vi "Fetch Power Measurement List Mode.vi"(6 "Step Index (1)":i32=1, 7 "Detector Type (RMS)":i32(ring) items=["RMS", "Minimum", "Maximum"], 8 "error in (no error)":errorcluster, 9 "Result Type (Current)":i32(ring) items=["Current", "Average", "Peak"], 10 "Instance (1)":i32=1, 11 "VISA resource name":refnum<visa-resource-name>) -> (0 "error out":errorcluster, 1 "Power":dbl format="%^.3e", 2 "Reliability":i32, 3 "VISA resource name out":refnum<visa-resource-name>)   [LabVIEW 2020, in "Rohde&Schwarz CMXP GPRF.lvlib"]
doc: "Returns the results of the GPRF power measurement for single step and \"Statistic\" evaluation mode. Initiate measurement first with VI rscmwgprf_PwrMeasInit.\n\nAttribute:\n-\n\nRemote-control commands:\nFETCh:GPRF:MEAS<i>:POWer:LIST:CURRent?\nFETCh:GPRF:MEAS<i>:POWer:LIST:MAXimum:CURRent?\nFETCh:GPRF:MEAS<i>:POWer:LIST:MINimum:CURRent?\nFETCh:GPRF:MEAS<i>:POWer:LIST:AVERage?\nFETCh:GPRF:MEAS<i>:POWer:LIST:PEAK:MAXimum?\nFETCh:GPRF:MEAS<i>:POWer:LIST:PEAK:MINimum?"
uses:
  <instrlib>/Rohde&Schwarz CMXP GPRF/Rohde&Schwarz CMXP GPRF.lvlib
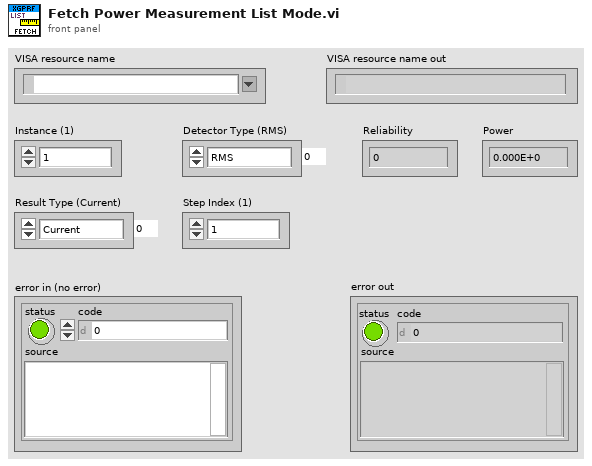
[diagram p1: front panel]
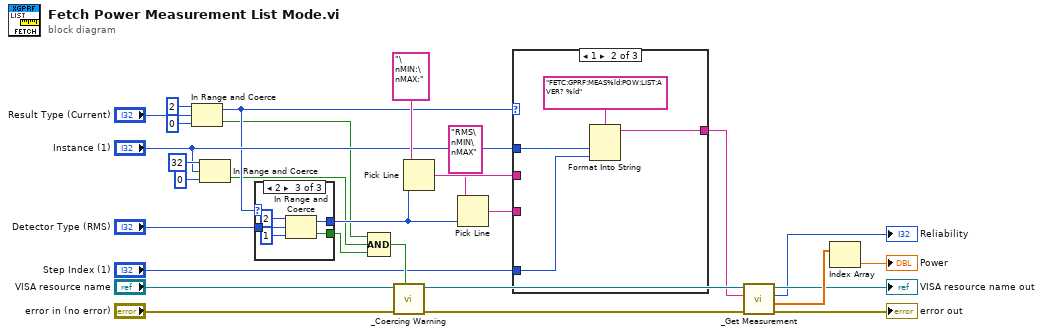
[diagram p0: block diagram]
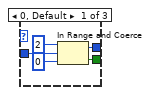
[diagram p2: hidden frame]
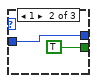
[diagram p3: hidden frame]
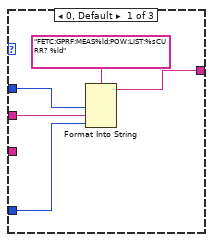
[diagram p4: hidden frame]
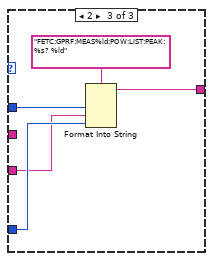
[diagram p5: hidden frame]
diagram:
  n1 = In Range and Coerce(upper limit=2, x="Result Type (Current)", lower limit=0) -> (coerced(x)=w5:i32, In Range?=w2:bool)
  n2 = In Range and Coerce(upper limit=32, x="Instance (1)", lower limit=0) -> (In Range?=w3:bool)  [unwired: 1 out]
  n3 = case shown="2" w5 {
    tunnel: [w31 TRUE w38] -> w4
    tunnel: [w30 w34 w37] -> w8
    tunnel: "Detector Type (RMS)" -> [w29 w34 w36]
    frame 0, Default {
      n4 = In Range and Coerce(upper limit=2, x=w29, lower limit=0) -> (coerced(x)=w30:i32, In Range?=w31:bool)
    }
    frame 1 {
    }
    frame 2 {
      n5 = In Range and Coerce(upper limit=2, x=w36, lower limit=1) -> (coerced(x)=w37:i32, In Range?=w38:bool)
    }
  }
  n6 = Compound Arithmetic op=AND(w2, w3, w4) -> (w24:bool)
  n7 = call <instrlib>:"_Coercing Warning.vi"("In Range?"=w24, "error in (no error)"="error in (no error)", "VISA resource name"="VISA resource name") -> ("error out"=w20:errorcluster, "VISA resource name out"=w21:refnum<visa-resource-name>)  [unwired: 7 in]
  n8 = Pick Line(multi-line string="\nMIN:\nMAX:", line index=w8) -> (output string=w25:string)  [unwired: 1 in]
  n9 = Pick Line(multi-line string="RMS\nMIN\nMAX", line index=w8) -> (output string=w9:string)  [unwired: 1 in]
  n10 = case shown="1" w5 {
    tunnel: w25 -> [w44 _ _]
    tunnel: "Instance (1)" -> [w42 w48 w52]
    tunnel: [w43 w47 w53] -> w1
    tunnel: "Step Index (1)" -> [w41 w46 w51]
    tunnel: w9 -> [_ _ w50]
    frame 0, Default {
      n11 = Format Into String(format string="FETC:GPRF:MEAS%ld:POW:LIST:%sCURR? %ld", w42, w44, w41) -> (resulting string=w43:string)  [unwired: 2 in, 1 out]
    }
    frame 1 {
      n12 = Format Into String(format string="FETC:GPRF:MEAS%ld:POW:LIST:AVER? %ld", w48, w46) -> (resulting string=w47:string)  [unwired: 2 in, 1 out]
    }
    frame 2 {
      n13 = Format Into String(format string="FETC:GPRF:MEAS%ld:POW:LIST:PEAK:%s? %ld", w52, w50, w51) -> (resulting string=w53:string)  [unwired: 2 in, 1 out]
    }
  }
  n14 = call <instrlib>:"_Get Measurement.vi"("error in (no error)"=w20, "Command"=w1, "VISA resource name"=w21) -> ("error out"=→"error out":errorcluster, "Data"=w19:dbl[], "Reliability"=→"Reliability":i32, "VISA resource name out"=→"VISA resource name out":refnum<visa-resource-name>)  [unwired: 5 in]
  n15 = Index Array(array=w19) -> (element=→"Power":dbl)  [unwired: 1 in]
